vi "MFLI disable Scope mode.vi"(10 "scopeModHandle in":T2 {"ModHandle" format="0x%08x"; "Conn" format="0x%08x"}, 11 "Lock-in Handle":T1 {"Handle" format="0x%08x"; "Conn" format="0x%08x"}) -> (3 "Handle Out":T1 {"Handle" format="0x%08x"; "Conn" format="0x%08x"})   [LabVIEW 2022 SP3, in "Lock-in module.lvlib"]
uses:
  Lock-in module.lvlib
  <instrlib>/Zurich Instruments LabOne/Public/Modules/ziTypeModHandle.ctl
  <instrlib>/Zurich Instruments LabOne/Public/ziTypeHandle.ctl
  <instrlib>/Zurich Instruments LabOne/Public/Configure/ziSetValueDoubleArray.vi
  <instrlib>/Zurich Instruments LabOne/Zurich Instruments LabOne.lvlib
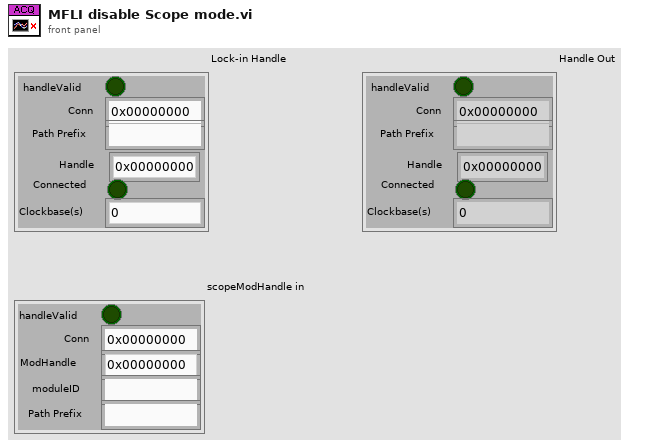
[diagram p1: front panel]
types:
  T1 = typedef "Zurich Instruments LabOne.lvlib/ziTypeHandle.ctl" = cluster{"handleValid":bool, "Conn":u64, "Path Prefix":string, "Handle":u64, "Connected":bool, "Clockbase(s)":dbl}
  T2 = typedef "Zurich Instruments LabOne.lvlib/ziTypeModHandle.ctl" = cluster{"handleValid":bool, "Conn":u64, "ModHandle":u64, "moduleID":string, "Path Prefix":string}
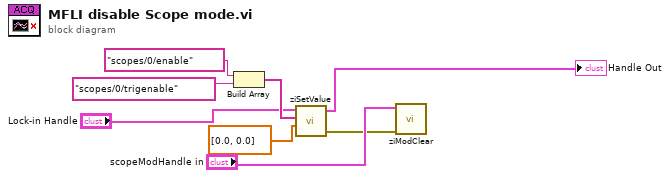
[diagram p0: block diagram]
diagram:
  n1 = Build Array("scopes/0/enable", "scopes/0/trigenable") -> (w6:string[])
  n2 = call-poly <instrlib>:"ziSetValue.vi"("Values"=dbl[] [0.0, 0.0] ("Value"), "Paths"=w6, "Handle In"="Lock-in Handle") -> ("Error Out"=w5:errorcluster, "Handle Out"=→"Handle Out":T1)  [unwired: 2 in]
  n3 = call <instrlib>:"ziModClear.vi"("Error In"=w5, "ziModHandle In"="scopeModHandle in") -> ()  [unwired: 7 in, 2 out]
